vi "GDSAPI_Example_AddDesignPattern.vi"() -> ()   [LabVIEW 2012]
uses:
  <resource>/Framework/Providers/Open_GDS/API/GDSAPI_SubVIs/GDSAPI_ClassProviderType.ctl
  <resource>/Framework/Providers/Open_GDS/API/GDSAPI_CreateClassType.ctl
  <resource>/Framework/Providers/Open_GDS/API/GDSAPI_SubVIs/GDSAPI_ClassTemplateType.ctl
  <resource>/Framework/Providers/Open_GDS/ClassProviders/Common/String/GDSString_MethodDescriptionType.ctl
  <resource>/Framework/Providers/Open_GDS/ClassProviders/Common/CommonVIs/CommonVIs_AttributeType.ctl
  <resource>/Framework/Providers/Open_GDS/ClassProviders/Common/CommonVIs/CommonVIs_AttributeDataType.ctl
  <resource>/Framework/Providers/Open_GDS/ClassProviders/Common/String/GDSString_AccessScopeModifierType.ctl
  <resource>/Framework/Providers/Open_GDS/ClassProviders/Common/String/GDSString_ModifierType.ctl
  <resource>/Framework/Providers/Open_GDS/ClassProviders/Common/CommonVIs/CommonVIs_PropertyType.ctl
panel:
  out "error out":errorcluster
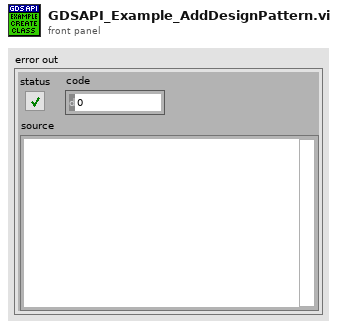
[diagram p1: front panel]
types:
  T1 = typedef "GDSString_MethodDescriptionType.ctl" = cluster{"ReturnType":T2, "MethodName":string, "AccessScope":T4, "Modifiers":T5[], "MethodDocumentation":string, "MethodContent":string, "MethodArguments":T2[], "GetProperty":T6, "SetProperty":T6}
  T2 = typedef "CommonVIs_AttributeType.ctl" = cluster{"Name":string, "DataType":T3, "ArrayDim":i32, "CtrlPath":path, "DataTypeString":string, "AccessScope":T4, "InitialData":variant}
  T3 = typedef "CommonVIs_AttributeDataType.ctl" = enum16{"UINT8", "INT8", "UINT16", "INT16", "UINT32", "INT32", "UINT64", "INT64", "SGL", "DBL", "EXT", "CSG", "CDB", "CXT", "TimeStamp", "STRING", "PATH", "BOOL", "ENUM", "RefNum", "VIRefNum", "LabVIEW Class", "Cluster", "Variant", "TypeDef", "Waveform", "LabVIEW Object", "Other", "void"}
  T4 = typedef "GDSString_AccessScopeModifierType.ctl" = enum16{"public", "private", "protected", "internal"}
  T5 = typedef "GDSString_ModifierType.ctl" = enum16{"abstract", "static", "final", "synchronized", "strictfp", "async", "const", "event", "extern", "new", "override", "partial", "readonly", "sealed", "unsafe", "virtual", "volatile"}
  T6 = typedef "CommonVIs_PropertyType.ctl" = cluster{"Active":bool, "AccessScope":T4, "Code":string}
  T7 = typedef "GDSAPI_ClassTemplateType.ctl" = enum16{"Standard", "Singleton", "Interface(By Aggregation)", "Interface(By VI Server)"}
  T8 = typedef "GDSAPI_CreateClassType.ctl" = cluster{"ClassProvider":T9, "NewClassFolder":path, "ParentLvClassFilePath":path, "ClassName":string, "ClassDescription":string, "ClassTemplate":T7}
  T9 = typedef "GDSAPI_ClassProviderType.ctl" = enum16{"LabVIEW Native(By value)", "GOOP-3(By reference)", "GOOP-4(By reference)"}
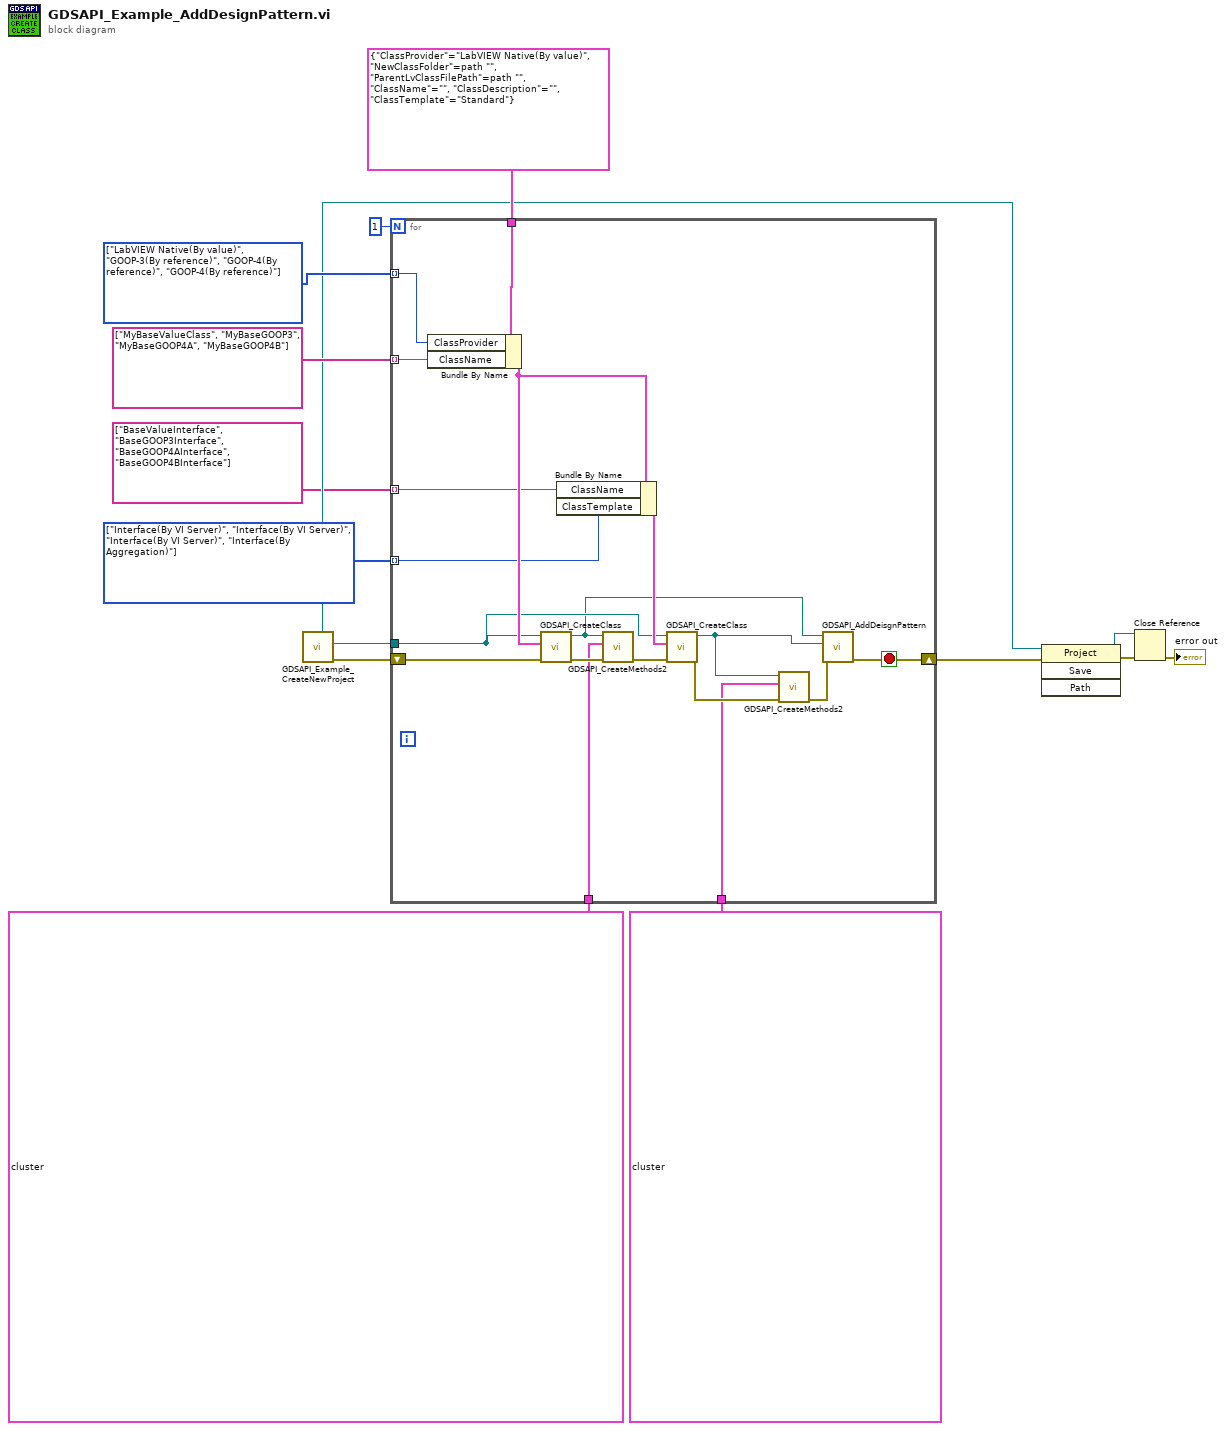
[diagram p0: block diagram]
diagram:
  w5 = T7[] [enum."Interface(By VI Server)", enum."Interface(By VI Server)", enum."Interface(By VI Server)", enum."Interface(By Aggregation)"] items=["Standard", "Singleton", "Interface(By Aggregation)", "Interface(By VI Server)"]
  w9 = T9[] [enum."LabVIEW Native(By value)", enum."GOOP-3(By reference)", enum."GOOP-4(By reference)", enum."GOOP-4(By reference)"] items=["LabVIEW Native(By value)", "GOOP-3(By reference)", "GOOP-4(By reference)"]
  n1 = call <resource>:"GDSAPI_Example_CreateNewProject.vi"() -> ("error out"=w15:errorcluster, "ProjectItem out"=w14:refnum<vi>, "ProjectRefOut"=w8:refnum<vi>)  [unwired: 8 in, 1 out]
  n2 = for {
    N: 1 -> [_]
    tunnel: w14 -> [w24]
    tunnel: T8 {"ClassProvider"=enum."LabVIEW Native(By value)", "NewClassFolder"=path "", "ParentLvClassFilePath"=path "", "ClassName"="", "ClassDescription"="", "ClassTemplate"=enum."Standard"} ("CreateClassType") -> [w33]
    tunnel: string[] ["MyBaseValueClass", "MyBaseGOOP3", "MyBaseGOOP4A", "MyBaseGOOP4B"] -> [w32] mode=indexing
    tunnel: w9 -> [w31] mode=indexing
    shift-right: [w29] -> w6
    shift-left: w15 -> [w30]
    tunnel: w5 -> [w26] mode=indexing
    tunnel: string[] ["BaseValueInterface", "BaseGOOP3Interface", "BaseGOOP4AInterface", "BaseGOOP4BInterface"] -> [w23] mode=indexing
    tunnel: T1[] [{"ReturnType"={"Name"="Message", "DataType"=enum."STRING", "ArrayDim"=0, "CtrlPath"=path "", "DataTypeString"="", "AccessScope"=enum."public", "InitialData"=variant}, "MethodName"="GetMessage", "AccessScope"=enum."public", "Modifiers"=[], "MethodDocumentation"="Doc Doc", "MethodContent"="static void Main()\n{\n    foreach (int number in SomeNumbers())\n    {\n        Console.Write(number.ToString() + \" \");\n    }\n    // Output: 3 5 8\n    Console.ReadKey();\n}", "MethodArguments"=[{"Name"="Get", "DataType"=enum."BOOL", "ArrayDim"=0, "CtrlPath"=path "", "DataTypeString"="", "AccessScope"=enum."public", "InitialData"=variant}], "GetProperty"={"Active"=FALSE, "AccessScope"=enum."public", "Code"=""}, "SetProperty"={"Active"=FALSE, "AccessScope"=enum."public", "Code"=""}}, {"ReturnType"={"Name"="Message", "DataType"=enum."STRING", "ArrayDim"=0, "CtrlPath"=path "", "DataTypeString"="", "AccessScope"=enum."public", "InitialData"=variant}, "MethodName"="GetMessage", "AccessScope"=enum."public", "Modifiers"=[], "MethodDocumentation"="Doc Doc", "MethodContent"="static void Main()\n{\n    foreach (int number in SomeNumbers())\n    {\n        Console.Write(number.ToString() + \" \");\n    }\n    // Output: 3 5 8\n    Console.ReadKey();\n}", "MethodArguments"=[{"Name"="Get", "DataType"=enum."BOOL", "ArrayDim"=0, "CtrlPath"=path "", "DataTypeString"="", "AccessScope"=enum."public", "InitialData"=variant}], "GetProperty"={"Active"=FALSE, "AccessScope"=enum."public", "Code"=""}, "SetProperty"={"Active"=FALSE, "AccessScope"=enum."public", "Code"=""}}] ("Methods") -> [w21]
    tunnel: T1[] [{"ReturnType"={"Name"="Number", "DataType"=enum."DBL", "ArrayDim"=0, "CtrlPath"=path "", "DataTypeString"="", "AccessScope"=enum."public", "InitialData"=variant}, "MethodName"="Do", "AccessScope"=enum."public", "Modifiers"=[], "MethodDocumentation"="My Doc", "MethodContent"=" public int Inventory\n  {\n    get\n    {\n       return _int;\n    }\n    set\n    {\n       // Just to make sure that if there is an increase in inventory then only we are notifying \n          the observers.\n          if (value > _int)\n             Notify();\n          _int = value;\n    }\n  }", "MethodArguments"=[{"Name"="A", "DataType"=enum."UINT8", "ArrayDim"=0, "CtrlPath"=path "", "DataTypeString"="", "AccessScope"=enum."public", "InitialData"=variant}, {"Name"="B", "DataType"=enum."UINT64", "ArrayDim"=1, "CtrlPath"=path "", "DataTypeString"="", "AccessScope"=enum."public", "InitialData"=variant}, {"Name"="C", "DataType"=enum."PATH", "ArrayDim"=0, "CtrlPath"=path "", "DataTypeString"="", "AccessScope"=enum."public", "InitialData"=variant}], "GetProperty"={"Active"=FALSE, "AccessScope"=enum."public", "Code"=""}, "SetProperty"={"Active"=FALSE, "AccessScope"=enum."public", "Code"=""}}] ("Methods") -> [w18]
    stop <- w29 stop-if-true
    n3 = Bundle By Name(cluster=w33, "ClassProvider"=w31, "ClassName"=w32) -> (w27:T8)
    n4 = call <resource>:"GDSAPI_CreateClass.vi"("error in (no error)"=w30, "CreateClassType"=w27, "ProjectItem"=w24) -> ("error out"=w28:errorcluster, "LvClassFileOut"=w16:path)  [unwired: 6 in, 1 out]
    n5 = Bundle By Name(cluster=w27, "ClassName"=w23, "ClassTemplate"=w26) -> (w25:T8)
    n6 = call <resource>:"GDSAPI_CreateMethods2.vi"("error in (no error)"=w28, "Methods"=w21, "ClassPath(*.lvclass)"=w16) -> ("error out"=w22:errorcluster)  [unwired: 8 in]
    n7 = call <resource>:"GDSAPI_CreateClass.vi"("error in (no error)"=w22, "CreateClassType"=w25, "ProjectItem"=w24) -> ("error out"=w20:errorcluster, "LvClassFileOut"=w17:path)  [unwired: 6 in, 1 out]
    n8 = call <resource>:"GDSAPI_CreateMethods2.vi"("error in (no error)"=w20, "Methods"=w18, "ClassPath(*.lvclass)"=w17) -> ("error out"=w19:errorcluster)  [unwired: 8 in]
    n9 = call <resource>:"GDSAPI_AddDeisgnPattern.vi"("error in (no error)"=w19, "InterfaceClass(*.lvclass)"=w17, "ClassPath(*.lvclass)"=w16) -> ("error out"=w29:errorcluster)  [unwired: 8 in]
  }
  n10 = invoke class="Project" method="Save"(reference=w8, error in=w6) -> (reference out=w12:refnum<vi>, error out=w13:errorcluster)  [unwired: 2 in, 2 out]
  n11 = Close Reference(reference=w12, error in (no error)=w13) -> (error out=→"error out":errorcluster)
